vi "CB Augment Controller Input Error.vi"(11 "K (gain matrix)":T1) -> (3 "K augmented":T1)   [LabVIEW 2020]
uses:
  <vilib>/Analysis/Matrix/Datatypes/RealMatrix.ctl
  <vilib>/Analysis/Matrix/NI_Matrix.lvlib
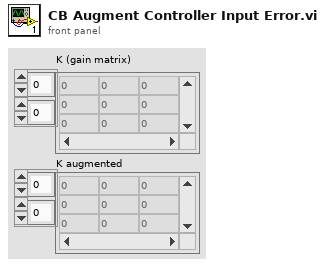
[diagram p1: front panel]
types:
  T1 = typedef "NI_Matrix.lvlib/RealMatrix.ctl" = dbl[][]
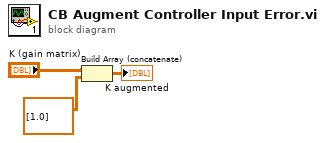
[diagram p0: block diagram]
diagram:
  n1 = Build Array (concatenate)("K (gain matrix)", T1 [[1.0]] ("array")) -> (→"K augmented":T1)
